vi "to string 1.0.vi"(8 "error in (no error)":errorcluster, 11 "Report Config.lvclass in":refnum<class "Report Config.lvclass">) -> (0 "error out":errorcluster, 2 "wrapped data":string, 3 "Report Config.lvclass out":refnum<class "Report Config.lvclass">)   [LabVIEW 2015, in "Report Config.lvclass"]
uses:
  Report Config.lvclass
  Report Config.lvclass/Report Config.ctl
  Report Formatters/Base Class/Config/Formatter Config.lvclass
  <vilib>/NI/Configuration Framework/serializable configuration/NISE_CEF_serializable configuration.lvclass
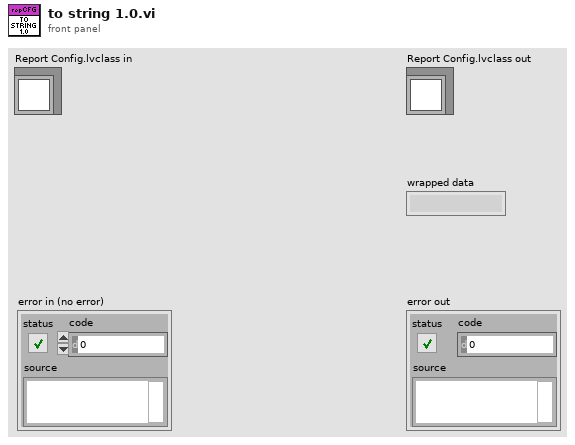
[diagram p1: front panel]
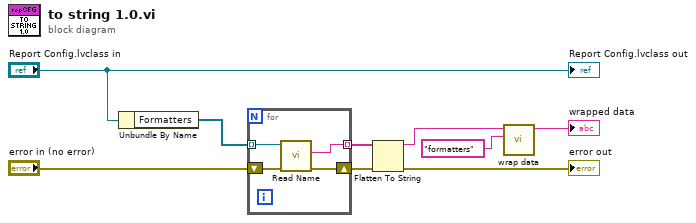
[diagram p0: block diagram]
diagram:
  n1 = Unbundle By Name("Report Config.lvclass in") -> ("Formatters"=w1:refnum<class "Formatter Config.lvclass">[])
  n2 = for {
    shift-right: [w13] -> w7
    shift-left: "error in (no error)" -> [w12]
    tunnel: w1 -> [w11] mode=indexing
    tunnel: [w10] -> w9 mode=indexing
    n3 = call-dynamic "Read Name.vi"("error in (no error)"=w12, "Formatter Config in"=w11) -> ("error out"=w13:errorcluster, "Name"=w10:string)  [unwired: 7 in, 1 out]
  }
  n4 = Flatten To String(anything=w9, error in (no error)=w7) -> (data string=w4:string, error out=→"error out":errorcluster)  [unwired: 2 in, 1 out]
  n5 = call <vilib>:"wrap data.vi"("identifier"="formatters", "data to wrap"=w4) -> ("wrapped data"=→"wrapped data":string)  [unwired: 9 in]
  "Report Config.lvclass out" <- "Report Config.lvclass in"
